vi "Gear.vi"(10 "Gear1?":bool, 11 "Gear0?":bool) -> ()   [LabVIEW 2016]
uses:
  <vilib>/Rock Robotics/WPI/Solenoid/WPI_SolenoidValue.ctl
  <vilib>/Rock Robotics/WPI/Solenoid/WPI_SolenoidSetEnum.vi
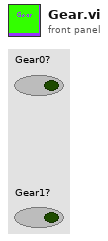
[diagram p1: front panel]
types:
  T1 = typedef "WPI_SolenoidValue.ctl" = enum16{"Off", "On", "Forward", "Reverse"}
  T2 = typedef "WPI_SolenoidDevRef.ctl" = cluster{"DevStatus":errorcluster, "Pneumatics Control Module":u8, "Forward Solenoid Channel":T3, "Reverse Solenoid Channel":T3}
  T3 = typedef "WPI_SolenoidChannel.ctl" = enum8{"Solenoid 0", "Solenoid 1", "Solenoid 2", "Solenoid 3", "Solenoid 4", "Solenoid 5", "Solenoid 6", "Solenoid 7", "Invalid"}
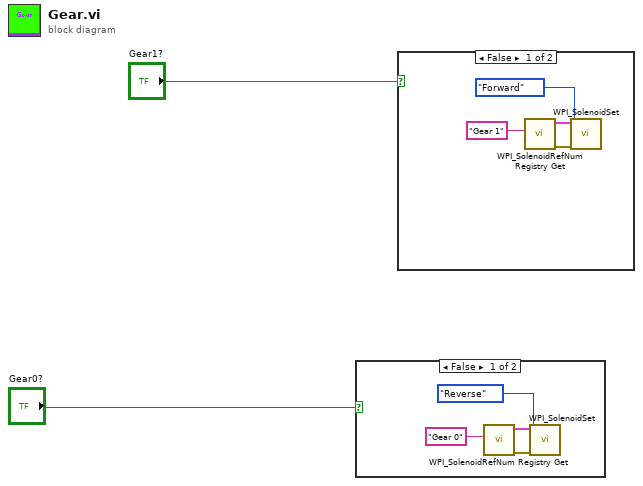
[diagram p0: block diagram]
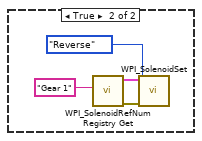
[diagram p2: hidden frame]
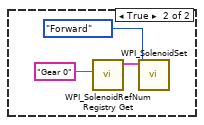
[diagram p3: hidden frame]
diagram:
  n1 = case shown="False" "Gear0?" {
    frame False {
      n2 = call <vilib>:"WPI_SolenoidRefNum Registry Get.vi"("refnum name"="Gear 0") -> ("error out"=w6:errorcluster, "SolenoidDevRef"=w5:T2)  [unwired: 9 in]
      n3 = call-poly <vilib>:"WPI_SolenoidSet.vi"("error in (no error)"=w6, "Value"=WPI_SolenoidValue."Reverse", "SolenoidDevRef"=w5) -> ()  [unwired: 7 in, 2 out]
    }
    frame True {
      n4 = call <vilib>:"WPI_SolenoidRefNum Registry Get.vi"("refnum name"="Gear 0") -> ("SolenoidDevRef"=w9:T2)  [unwired: 9 in, 1 out]
      n5 = call-poly <vilib>:"WPI_SolenoidSet.vi"("Value"=WPI_SolenoidValue."Forward", "SolenoidDevRef"=w9) -> ()  [unwired: 8 in, 2 out]
    }
  }
  n6 = case shown="False" "Gear1?" {
    frame False {
      n7 = call <vilib>:"WPI_SolenoidRefNum Registry Get.vi"("refnum name"="Gear 1") -> ("error out"=w10:errorcluster, "SolenoidDevRef"=w11:T2)  [unwired: 9 in]
      n8 = call-poly <vilib>:"WPI_SolenoidSet.vi"("error in (no error)"=w10, "Value"=WPI_SolenoidValue."Forward", "SolenoidDevRef"=w11) -> ()  [unwired: 7 in, 2 out]
    }
    frame True {
      n9 = call <vilib>:"WPI_SolenoidRefNum Registry Get.vi"("refnum name"="Gear 1") -> ("error out"=w17:errorcluster, "SolenoidDevRef"=w16:T2)  [unwired: 9 in]
      n10 = call-poly <vilib>:"WPI_SolenoidSet.vi"("error in (no error)"=w17, "Value"=WPI_SolenoidValue."Reverse", "SolenoidDevRef"=w16) -> ()  [unwired: 7 in, 2 out]
    }
  }
